vi "SetJogStepSize.vi"(8 "error in (no error)":errorcluster, 10 "Jog Step Size":dbl, 11 "ThorlabsLabJack in":refnum<class "ThorlabsLabJack.lvclass">) -> (0 "error out":errorcluster, 3 "ThorlabsLabJack out":refnum<class "ThorlabsLabJack.lvclass">)   [LabVIEW 2018, in "ThorlabsLabJack.lvlib" / "ThorlabsLabJack.lvclass"]
uses:
  ThorlabsLabJack.lvclass
  ThorlabsLabJack.lvclass/ThorlabsLabJack.ctl
  C:/Projects/LabVIEW/In-Progress/Chetan Malpure/Axis/Thorlabs LabJack/Drivers/Thorlabs.MotionControl.IntegratedStepperMotorsCLI.dll
  Drivers/Thorlabs.MotionControl.IntegratedStepperMotorsCLI.dll
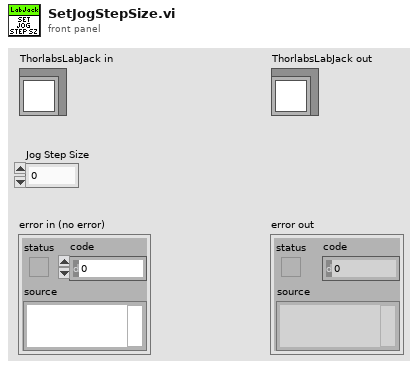
[diagram p1: front panel]
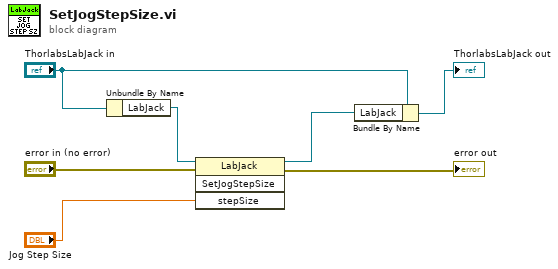
[diagram p0: block diagram]
diagram:
  n1 = Unbundle By Name("ThorlabsLabJack in") -> ("LabJack"=w5:refnum<k24>)
  n2 = invoke class="LabJack" method="SetJogStepSize"(reference=w5, error in="error in (no error)", "stepSize"="Jog Step Size") -> (reference out=w2:refnum<k24>, error out=→"error out":errorcluster)  [unwired: 1 in, 2 out]
  n3 = Bundle By Name(cluster="ThorlabsLabJack in", "LabJack"=w2) -> (→"ThorlabsLabJack out":refnum<class "ThorlabsLabJack.lvclass">)
